vi "Convert_From_Variant.vi"(8 "error in":errorcluster, 10 "Data in":T2) -> (0 "error out":errorcluster, 2 "String data out":string[](array[string]))   [LabVIEW 2023]
uses:
  Controls/redis-reply.ctl
  From OpenG-VariantDataLibrary/Type Descriptor Enumeration.ctl
panel:
  out "Array":T1[](array[typedef]) format="%.0x"
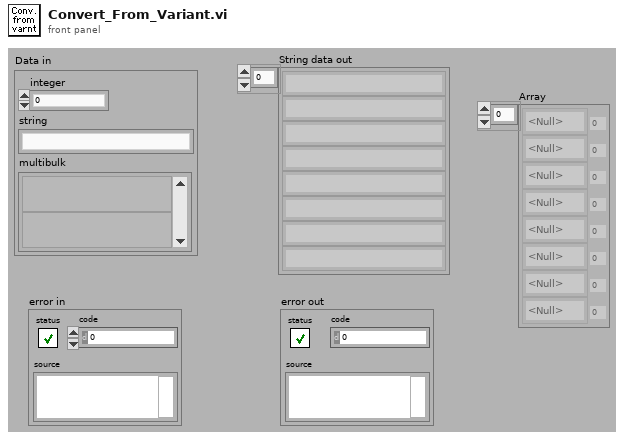
[diagram p1: front panel]
types:
  T1 = typedef "Type Descriptor Enumeration.ctl" = enum8{"<Null>", "I8", "I16", "I32", "I64", "U8", "U16", "U32", "U64", "SGL", "DBL", "EXT", "CSG", "CDB", "CXT", "0x0F", "0x10", "0x11", "0x12", "0x13", "0x14", "Enum U8", "Enum U16", "Enum U32", "Enum U64", "SGL PQ", "DBL PQ", "EXT PQ", "CSG PQ", "CDB PQ", "CXT PQ", "0x1F", "0x20", "Boolean", "0x22", "0x23", "0x24", "0x25", "0x26", "0x27", "0x28", "0x29", "0x2A", "0x2B", "0x2C", "0x2D", "0x2E", "0x2F", "String", "0x31", "Path", "Pict", "0x34", "0x35", "0x36", "DAQ", "0x38", "0x39", "0x3A", "0x3B", "0x3C", "0x3D", "0x3E", "0x3F", "Array", "0x41", "0x42", "0x43", "0x44", "0x45", "0x46", "0x47", "0x48", "0x49", "0x4A", "0x4B", "0x4C", "0x4D", "0x4E", "0x4F", "Cluster", "0x51", "0x52", "Variant", "Waveform", "0x55", "0x56", "0x57", "0x58", "0x59", "0x5A", "0x5B", "0x5C", "0x5D", "0x5E", "Fixed Point", "0x60", "0x61", "0x62", "0x63", "0x64", "0x65", "0x66", "0x67", "0x68", "0x69", "0x6A", "0x6B", "0x6C", "0x6D", "0x6E", "0x6F", "Refnum", "0x71", "0x72", "Set Collection", "Map Collection"}
  T2 = typedef "redis-reply.ctl" = cluster{"integer":i64, "string":string, "multibulk":variant[]}
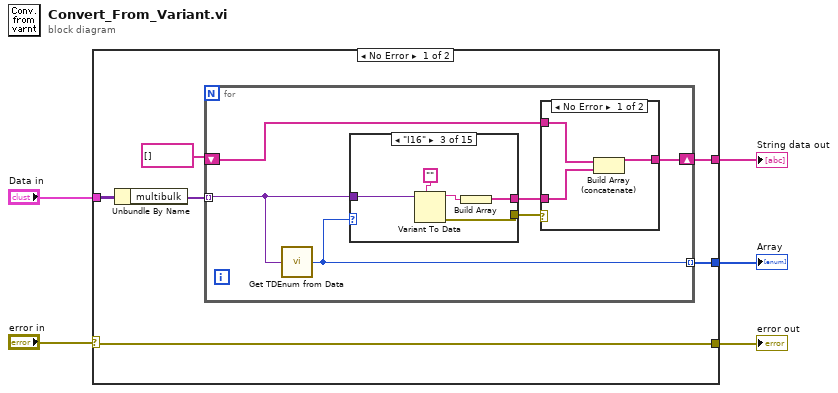
[diagram p0: block diagram]
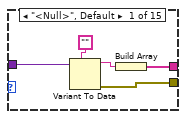
[diagram p2: hidden frame]
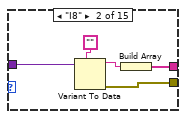
[diagram p3: hidden frame]
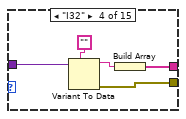
[diagram p4: hidden frame]
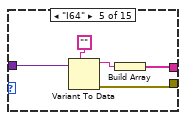
[diagram p5: hidden frame]
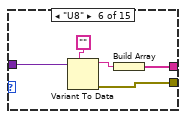
[diagram p6: hidden frame]
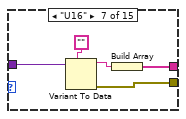
[diagram p7: hidden frame]
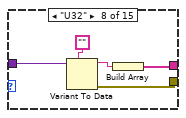
[diagram p8: hidden frame]
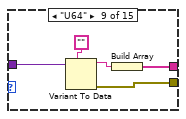
[diagram p9: hidden frame]
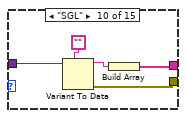
[diagram p10: hidden frame]
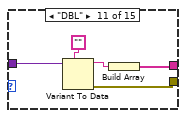
[diagram p11: hidden frame]
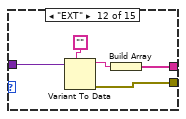
[diagram p12: hidden frame]
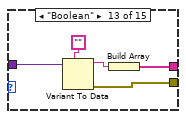
[diagram p13: hidden frame]
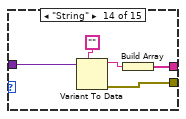
[diagram p14: hidden frame]
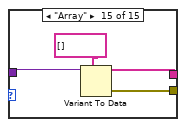
[diagram p15: hidden frame]
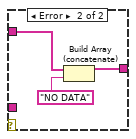
[diagram p16: hidden frame]
diagram:
  n1 = case shown="No Error" "error in" {
    selector: "error in" -> [w7 w98]
    tunnel: "Data in" -> [w9 _]
    tunnel: [w8 _] -> w3
    tunnel: [w7 w98] -> w5
    tunnel: [w6 _] -> w1
    frame No Error {
      n2 = Unbundle By Name(w9) -> ("multibulk"=w10:variant[])
      n3 = for {
        tunnel: w10 -> [w14] mode=indexing
        shift-right: [w16] -> w8
        shift-left: string[] [] -> [w17]
        tunnel: [w15] -> w6 mode=indexing
        n4 = call "Get TDEnum from Data.vi"("Data"=w14) -> ("Type Descriptor Enumeration"=w15:T1)  [unwired: 4 in]
        n5 = case shown="\"I16\"" w15 {
          tunnel: w14 -> [w18 w24 w28 w33 w38 w43 w48 w53 w58 w63 w68 w73 w78 w86 w88]
          tunnel: [w19 w23 w30 w34 w39 w44 w49 w54 w59 w64 w69 w74 w79 w85 w90] -> w13
          tunnel: [w20 w25 w29 w35 w40 w45 w50 w55 w60 w65 w70 w75 w80 w83 w89] -> w12
          frame "<Null>", Default {
            n6 = Variant To Data(type="", Variant=w18) -> (data=w22:string, error out=w19:errorcluster)  [unwired: 1 in]
            n7 = Build Array(w22) -> (w20:string[])
          }
          frame "I8" {
            n8 = Variant To Data(type="", Variant=w24) -> (data=w27:string, error out=w23:errorcluster)  [unwired: 1 in]
            n9 = Build Array(w27) -> (w25:string[])
          }
          frame "I16" {
            n10 = Variant To Data(type="", Variant=w28) -> (data=w31:string, error out=w30:errorcluster)  [unwired: 1 in]
            n11 = Build Array(w31) -> (w29:string[])
          }
          frame "I32" {
            n12 = Variant To Data(type="", Variant=w33) -> (data=w37:string, error out=w34:errorcluster)  [unwired: 1 in]
            n13 = Build Array(w37) -> (w35:string[])
          }
          frame "I64" {
            n14 = Variant To Data(type="", Variant=w38) -> (data=w41:string, error out=w39:errorcluster)  [unwired: 1 in]
            n15 = Build Array(w41) -> (w40:string[])
          }
          frame "U8" {
            n16 = Variant To Data(type="", Variant=w43) -> (data=w47:string, error out=w44:errorcluster)  [unwired: 1 in]
            n17 = Build Array(w47) -> (w45:string[])
          }
          frame "U16" {
            n18 = Variant To Data(type="", Variant=w48) -> (data=w51:string, error out=w49:errorcluster)  [unwired: 1 in]
            n19 = Build Array(w51) -> (w50:string[])
          }
          frame "U32" {
            n20 = Variant To Data(type="", Variant=w53) -> (data=w57:string, error out=w54:errorcluster)  [unwired: 1 in]
            n21 = Build Array(w57) -> (w55:string[])
          }
          frame "U64" {
            n22 = Variant To Data(type="", Variant=w58) -> (data=w61:string, error out=w59:errorcluster)  [unwired: 1 in]
            n23 = Build Array(w61) -> (w60:string[])
          }
          frame "SGL" {
            n24 = Variant To Data(type="", Variant=w63) -> (data=w67:string, error out=w64:errorcluster)  [unwired: 1 in]
            n25 = Build Array(w67) -> (w65:string[])
          }
          frame "DBL" {
            n26 = Variant To Data(type="", Variant=w68) -> (data=w71:string, error out=w69:errorcluster)  [unwired: 1 in]
            n27 = Build Array(w71) -> (w70:string[])
          }
          frame "EXT" {
            n28 = Variant To Data(type="", Variant=w73) -> (data=w77:string, error out=w74:errorcluster)  [unwired: 1 in]
            n29 = Build Array(w77) -> (w75:string[])
          }
          frame "Boolean" {
            n30 = Variant To Data(type="", Variant=w78) -> (data=w81:string, error out=w79:errorcluster)  [unwired: 1 in]
            n31 = Build Array(w81) -> (w80:string[])
          }
          frame "String" {
            n32 = Variant To Data(type="", Variant=w86) -> (data=w84:string, error out=w85:errorcluster)  [unwired: 1 in]
            n33 = Build Array(w84) -> (w83:string[])
          }
          frame "Array" {
            n34 = Variant To Data(type=string[] [], Variant=w88) -> (data=w89:string[], error out=w90:errorcluster)  [unwired: 1 in]
          }
        }
        n35 = case shown="No Error" w13 {
          tunnel: w12 -> [w93 _]
          tunnel: w17 -> [w94 w97]
          tunnel: [w92 w96] -> w16
          frame No Error {
            n36 = Build Array (concatenate)(w94, w93) -> (w92:string[])
          }
          frame Error {
            n37 = Build Array (concatenate)(w97, "NO DATA") -> (w96:string[])
          }
        }
      }
    }
    frame Error {
    }
  }
  "String data out" <- w3
  "error out" <- w5
  "Array" <- w1
